vi "Dequeue.vi"(8 "error in":errorcluster) -> (0 "error out":errorcluster, 2 "Data":variant, 3 "State":T1)   [LabVIEW 2018, in "IO.lvclass"]
uses:
  IO.lvclass
  State.ctl
  Queue Data.ctl
panel:
  out "# elements in queue":i32
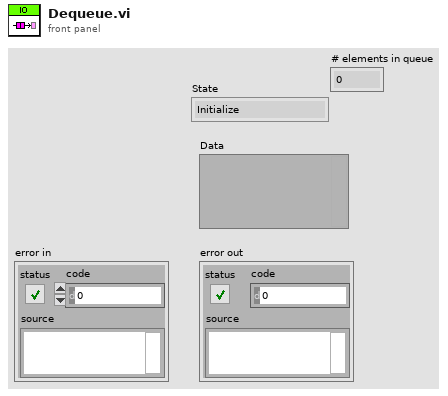
[diagram p1: front panel]
types:
  T1 = typedef "IO.lvclass/State.ctl" = enum16{"Initialize", "GlobalConfig", "ESTOP", "Abort", "S1Ouputs", "S2Outputs", "S3Ouputs", "S4Outputs", "S5Outputs", "S6Outputs", "Read", "Error", "Exit"}
  T2 = typedef "IO.lvclass/Queue Data.ctl" = cluster{"State":T1, "Data":variant}
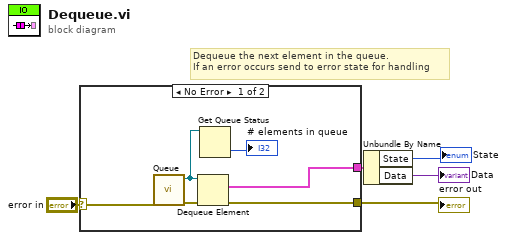
[diagram p0: block diagram]
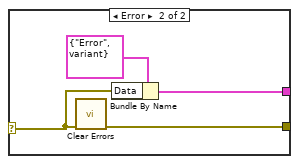
[diagram p2: hidden frame]
diagram:
  # "Dequeue the next element in the queue. \nIf an error occurs send to error state for handling"
  n1 = case shown="No Error" "error in" {
    selector: "error in" -> [w11 w13]
    tunnel: [w9 w15] -> w2
    tunnel: [w8 w12] -> w3
    frame No Error {
      n2 = call "Queue.vi"("error in"=w11) -> ("error out"=w10:errorcluster, "queue out"=w7:refnum<queue>)  [unwired: 9 in]
      n3 = Dequeue Element(queue=w7, error in (no error)=w10) -> (element=w8:T2, error out=w9:errorcluster)  [unwired: 1 in, 2 out]
      n4 = Get Queue Status(queue=w7) -> (# elements in queue=→"# elements in queue":i32)  [unwired: 2 in, 7 out]
    }
    frame Error {
      n5 = call <vilib>:"Clear Errors.vi"("error in (no error)"=w13) -> ("error out"=w15:errorcluster)  [unwired: 5 in, 1 out]
      n6 = Bundle By Name(cluster=T2 {"State"=enum."Error", "Data"=variant}, "Data"=w13) -> (w12:T2)
    }
  }
  "error out" <- w2
  n7 = Unbundle By Name(w3) -> ("State"=→"State":T1, "Data"=→"Data":variant)
